vi "to string.vi"(8 "error in":errorcluster, 11 "channel in":refnum<class "Modbus Module Channel.lvclass">) -> (0 "error out":errorcluster, 1 "channel data":string, 2 "identifier":string, 3 "channel out":refnum<class "Modbus Module Channel.lvclass">)   [LabVIEW 2015, in "Modbus Module Channel.lvclass"]
doc: "NI Tag Bus Module Framework 1.0.2.36\nNI Systems Engineering"
uses:
  Modbus Module Channel.lvclass
  Modbus Module Channel.lvclass/Modbus Module Channel.ctl
  <vilib>/NI/Tag Bus Module Framework/channel/TBM channel.lvclass
  <vilib>/NI/Configuration Framework/serializable configuration/NISE_CEF_serializable configuration.lvclass
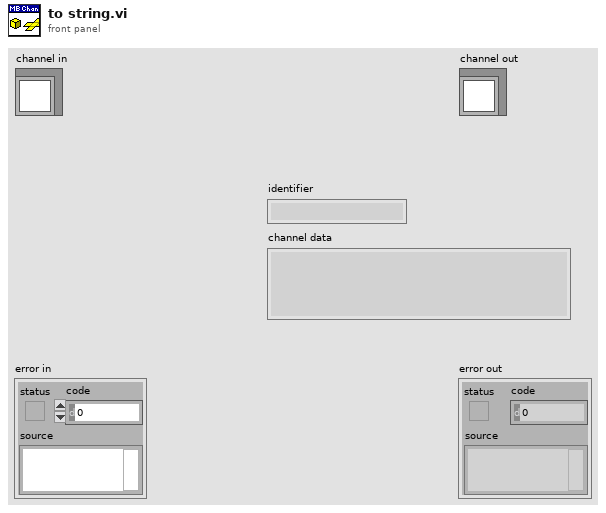
[diagram p1: front panel]
types:
  T1 = typedef "Modbus Module Channel.lvclass/data bank type.ctl" = enum16{"Coils", "Discrete Inputs", "Input Registers", "Holding Registers"}
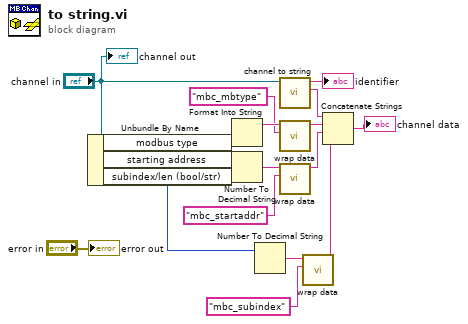
[diagram p0: block diagram]
diagram:
  n1 = Unbundle By Name("channel in") -> ("modbus type"=w12:T1, "starting address"=w11:u16, "subindex/len (bool/str)"=w1:i32)
  n2 = Format Into String(w12) -> (resulting string=w9:string)  [unwired: 3 in, 1 out]
  n3 = Number To Decimal String(number=w11) -> (decimal integer string=w10:string)  [unwired: 1 in]
  n4 = Number To Decimal String(number=w1) -> (decimal integer string=w3:string)  [unwired: 1 in]
  n5 = call <vilib>:"channel to string.vi"("channel in"="channel in") -> ("channel data"=w14:string, "identifier"=→"identifier":string)  [unwired: 9 in]
  n6 = call <vilib>:"wrap data.vi"("identifier"="mbc_mbtype", "data to wrap"=w9) -> ("wrapped data"=w5:string)  [unwired: 9 in]
  n7 = call <vilib>:"wrap data.vi"("identifier"="mbc_startaddr", "data to wrap"=w10) -> ("wrapped data"=w6:string)  [unwired: 9 in]
  n8 = call <vilib>:"wrap data.vi"("identifier"="mbc_subindex", "data to wrap"=w3) -> ("wrapped data"=w2:string)  [unwired: 9 in]
  n9 = Concatenate Strings(w14, w5, w6, w2) -> (→"channel data":string)
  "error out" <- "error in"
  "channel out" <- "channel in"
